vi "GetVacPressureAverage.vi"(3 "error in":errorcluster, 4 "timeout":dbl=1.0, 5 "Num Averages":i32=5, 6 "DAQmx Global Channel":refnum<k21>="USB-VacGapCG") -> (0 "Vac Gap Read Error":errorcluster, 1 "Run Time (ms)":u32, 2 "Vac Gap \nPressure (torr)":dbl=36.0610879504122 format="%0.2f")   [LabVIEW 2016]
uses:
  <vilib>/DAQmx/read.llb/DAQmx Read (Analog 2D DBL NChan NSamp).vi
  <vilib>/DAQmx/miscellaneous.llb/DAQmx Fill In Error Info.vi
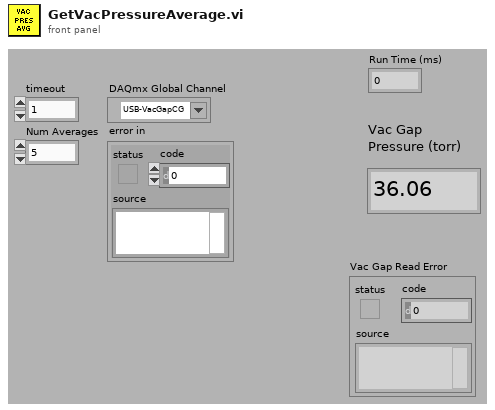
[diagram p1: front panel]
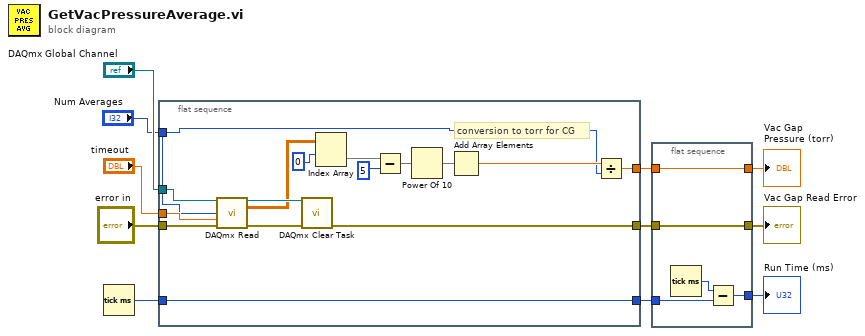
[diagram p0: block diagram]
diagram:
  n1 = Tick Count (ms)() -> (millisecond timer value=w7:u32)
  n2 = flat-sequence {
    tunnel: "DAQmx Global Channel" -> [w27]
    tunnel: "timeout" -> [w20]
    tunnel: "error in" -> [w19]
    tunnel: "Num Averages" -> [w16]
    tunnel: [w15] -> w4
    tunnel: [w14] -> w6
    tunnel: w7 -> [w13]
    tunnel: [w13] -> w2
    frame #0 {
      # "conversion to torr for CG"
      n3 = call-poly <vilib>:"DAQmx Read.vi"("task/channels in"=w27, "number of samples per channel"=w16, "timeout"=w20, "error in"=w19) -> ("task out"=w26:refnum<k21>, "data"=w22:dbl[][], "error out"=w25:errorcluster)  [unwired: 9 in]
      n4 = call <vilib>:"DAQmx Clear Task.vi"("task in"=w26, "error in"=w25) -> ("error out"=w14:errorcluster)  [unwired: 13 in]
      n5 = Index Array(array=w22, index (row)=0 ("disabled index (col)")) -> (element=w21:dbl[])  [unwired: 1 in]
      n6 = Subtract(x=w21, y=5) -> (x-y=w23:dbl[])
      n7 = Power Of 10(x=w23) -> (10^x=w18:dbl[])
      n8 = Add Array Elements(numeric array=w18) -> (sum=w17:dbl)
      n9 = Divide(x=w17, y=w16) -> (x/y=w15:dbl)
    }
  }
  n10 = flat-sequence {
    tunnel: w6 -> [w32]
    tunnel: [w32] -> w5
    tunnel: w4 -> [w31]
    tunnel: [w31] -> w3
    tunnel: w2 -> [w29]
    tunnel: [w28] -> w1
    frame #0 {
      n11 = Tick Count (ms)() -> (millisecond timer value=w30:u32)
      n12 = Subtract(x=w30, y=w29) -> (x-y=w28:u32)
    }
  }
  "Vac Gap \nPressure (torr)" <- w3
  "Vac Gap Read Error" <- w5
  "Run Time (ms)" <- w1
